vi "Remove User.vi"(0 "User Manager Model in":refnum<class "User Manager Model.lvclass">, 5 "Username":string, 11 "error in (no error)":errorcluster) -> (4 "User Manager Model out":refnum<class "User Manager Model.lvclass">, 15 "error out":errorcluster)   [LabVIEW 2017, in "User Manager Model.lvlib" / "User Manager Model.lvclass"]
uses:
  User Manager Model.lvclass
  C:/Program Files/National Instruments/LabVIEW 2017/vi.lib/ActorFramework/Actor/Actor.lvclass
  User Manager Model Messages/Get All Users Msg/Get All Users Msg.lvclass
  C:/Program Files/National Instruments/LabVIEW 2017/vi.lib/ActorFramework/Message/Message.lvclass
  User Manager Model Messages/Save Msg/Save Msg.lvclass
  <vilib>/ActorFramework/Actor/Actor.lvclass/Actor.ctl
  <vilib>/ActorFramework/Message Enqueuer/Message Enqueuer.lvclass/Message Enqueuer.ctl
  User Manager Model.lvclass/User Manager Model.ctl
  <vilib>/ActorFramework/Message Enqueuer/Init from Existing Queue.vi
  <vilib>/ActorFramework/Message Priority Queue/Priority Enqueue.vi
  <vilib>/ActorFramework/Message Enqueuer/Message Enqueuer.lvclass
  <vilib>/gpm_packages/@cs/user-manager/Source/User Configuration Manager Ref/By Ref.lvlib
  <vilib>/ActorFramework/Actor/Actor.lvclass
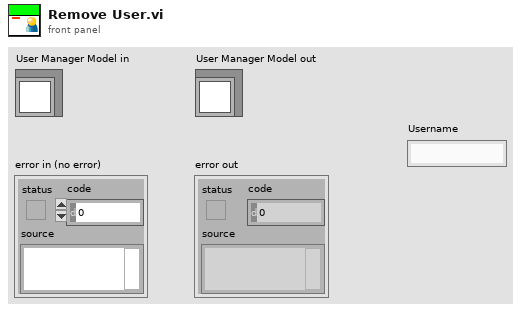
[diagram p1: front panel]
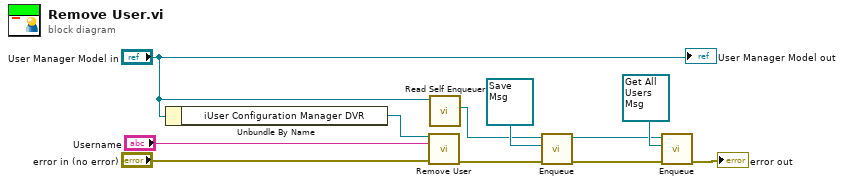
[diagram p0: block diagram]
diagram:
  n1 = Unbundle By Name("User Manager Model in") -> ("iUser Configuration Manager DVR"=w11:refnum<data-value>)
  n2 = call <vilib>:"Remove User.vi"("iUser Configuration Manager DVR"=w11, "Username"="Username", "error in"="error in (no error)") -> ("error out"=w5:errorcluster)  [unwired: 10 in, 2 out]
  n3 = call <vilib>:"Read Self Enqueuer.vi"("Actor"="User Manager Model in") -> ("Self Enqueuer"=w2:refnum<class "Message Enqueuer.lvclass">)  [unwired: 10 in]
  n4 = call <vilib>:"Enqueue.vi"("error in (no error)"=w5, "Message"=refnum<class "Save Msg.lvclass"> refnum ("User Manager Model.lvlib:Save Msg.lvclass"), "Message Enqueuer in"=w2) -> ("error out"=w4:errorcluster, "Message Enqueuer out"=w1:refnum<class "Message Enqueuer.lvclass">)  [unwired: 7 in]
  n5 = call <vilib>:"Enqueue.vi"("error in (no error)"=w4, "Message"=refnum<class "Get All Users Msg.lvclass"> refnum ("User Manager Model.lvlib:Get All Users Msg.lvclass"), "Message Enqueuer in"=w1) -> ("error out"=→"error out":errorcluster)  [unwired: 7 in, 1 out]
  "User Manager Model out" <- "User Manager Model in"
